vi "Poly Set Map Remove Type.vi"(7 "Poly Ref Map":T3, 8 "error in (no error)":errorcluster, 9 "Delete Files?":bool, 10 "Data Type to Remove":string[](array[string]), 11 "Poly Set Map in":T1) -> (0 "error out":errorcluster, 1 "Data Type Library Path":path, 2 "Data Type Directory":path, 3 "Poly Set Map out":T1)   [LabVIEW 2020]
uses:
  _td_map_PolyRef.ctl
  _td_map_PolyInstanceInfo.ctl
  _td_cluster_InstanceInfo.ctl
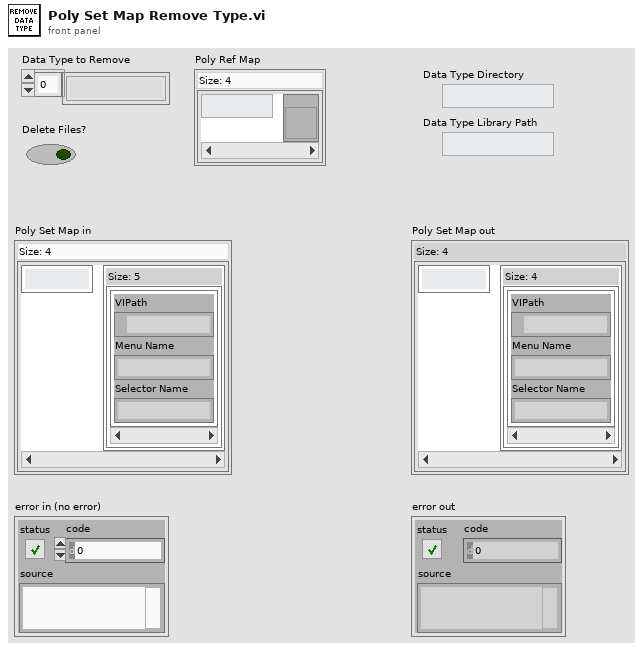
[diagram p1: front panel]
types:
  T1 = typedef "_td_map_PolyInstanceInfo.ctl" = map{string, set{T2}}
  T2 = typedef "_td_cluster_InstanceInfo.ctl" = cluster{"VIPath":path, "Menu Name":string, "Selector Name":string}
  T3 = typedef "_td_map_PolyRef.ctl" = map{string, refnum<vi>}
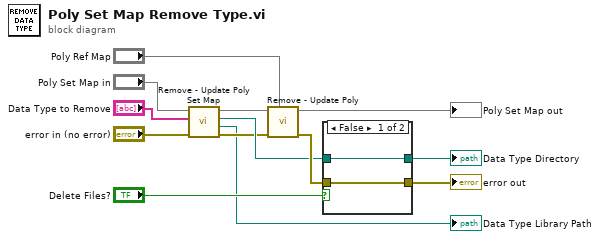
[diagram p0: block diagram]
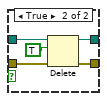
[diagram p2: hidden frame]
diagram:
  n1 = call "Remove - Update Poly Set Map.vi"("error in (no error)"="error in (no error)", "Data Type to Remove"="Data Type to Remove", "Poly Set Map in in"="Poly Set Map in") -> ("error out"=w5:errorcluster, "Data Type Library Path"=→"Data Type Library Path":path, "Data Type Directory"=w10:path, "Poly Set Map out"=w7:T1)  [unwired: 5 in]
  n2 = call "Remove - Update Poly.vi"("Poly Ref Map"="Poly Ref Map", "error in (no error)"=w5, "Poly Set Map in"=w7) -> ("error out"=w13:errorcluster, "Poly Set Map out"=→"Poly Set Map out":T1)  [unwired: 7 in]
  n3 = case shown="False" "Delete Files?" {
    tunnel: w10 -> [w14 w20]
    tunnel: [w15 w19] -> w8
    tunnel: w13 -> [w15 w18]
    tunnel: [w14 w16] -> w2
    frame False {
    }
    frame True {
      n4 = Delete(path (use dialog)=w20, entire hierarchy (F)=TRUE, error in=w18) -> (deleted path=w16:path, error out=w19:errorcluster)  [unwired: 2 in, 1 out]
    }
  }
  "error out" <- w8
  "Data Type Directory" <- w2
